vi "2022SignalManipulation.vi"(9 "Cold Junction Temp":dbl, 11 "Data":dbl[][](array[numeric])) -> (3 "Array":dbl[](array[numeric]))   [LabVIEW 2021]
panel:
  out "Array 3":dbl[](array[numeric])
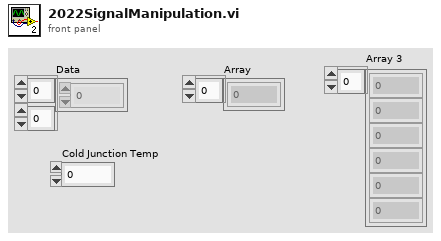
[diagram p1: front panel]
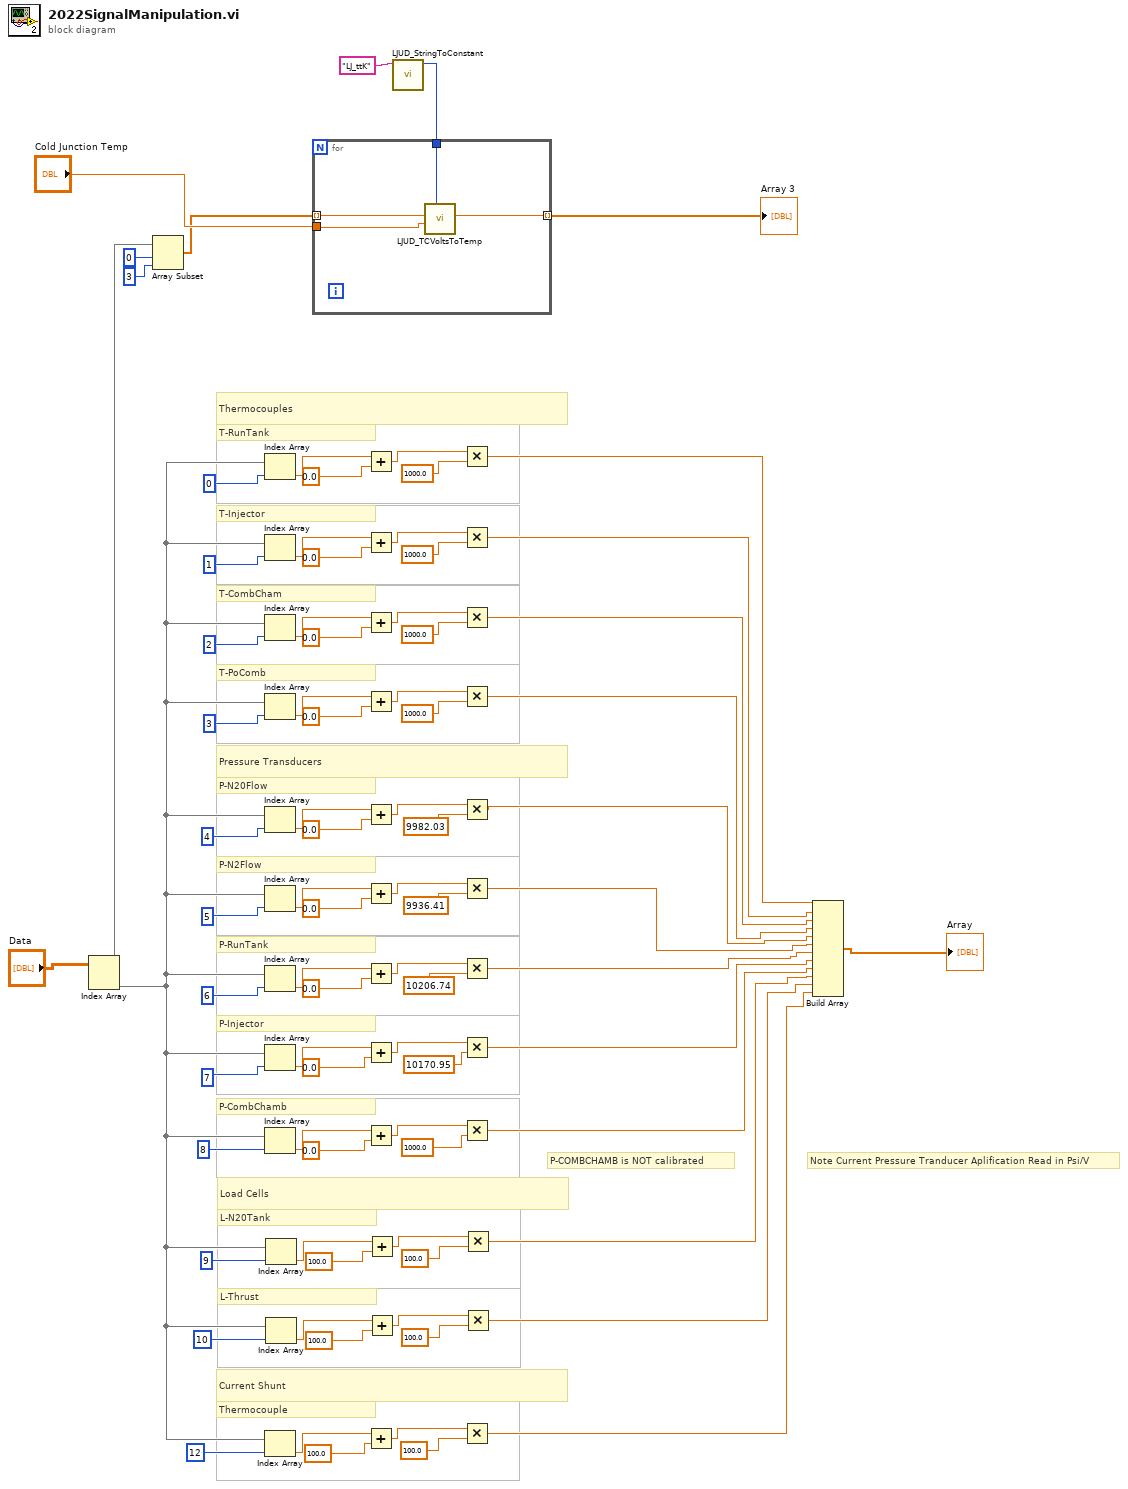
[diagram p0: block diagram]
diagram:
  # "P-COMBCHAMB is NOT calibrated"
  # "Note Current Pressure Tranducer Aplification Read in Psi/V"
  # "L-Thrust"
  # "Load Cells"
  # "L-N20Tank"
  # "P-CombChamb"
  # "Current Shunt"
  # "Thermocouple"
  # "P-Injector"
  # "P-RunTank"
  # "P-N2Flow"
  # "Pressure Transducers"
  # "P-N20Flow"
  # "T-PoComb"
  # "T-CombCham"
  # "T-Injector"
  # "Thermocouples"
  # "T-RunTank"
  n1 = Index Array(array="Data") -> (element=w16:dbl[])  [unwired: 2 in]
  n2 = Array Subset(array=w16, index=0, length=3) -> (w27:dbl[])
  n3 = Index Array(array=w16, index=0 ("index (col)")) -> (element=w57:dbl)
  n4 = Index Array(array=w16, index=1 ("index (col)")) -> (element=w56:dbl)
  n5 = Index Array(array=w16, index=2 ("index (col)")) -> (element=w55:dbl)
  n6 = Index Array(array=w16, index=3 ("index (col)")) -> (element=w54:dbl)
  n7 = Index Array(array=w16, index=4 ("index (col)")) -> (element=w53:dbl)
  n8 = Index Array(array=w16, index=5 ("index (col)")) -> (element=w52:dbl)
  n9 = Index Array(array=w16, index=6 ("index (col)")) -> (element=w51:dbl)
  n10 = Index Array(array=w16, index=7 ("index (col)")) -> (element=w50:dbl)
  n11 = Index Array(array=w16, index=8 ("index (col)")) -> (element=w47:dbl)
  n12 = Index Array(array=w16, index=12 ("index (col)")) -> (element=w44:dbl)
  n13 = Index Array(array=w16, index=9) -> (element=w18:dbl)
  n14 = Index Array(array=w16, index=10) -> (element=w17:dbl)
  n15 = Add(x=w57, y=0.0) -> (x+y=w82:dbl)
  n16 = Add(x=w56, y=0.0) -> (x+y=w79:dbl)
  n17 = Add(x=w55, y=0.0) -> (x+y=w76:dbl)
  n18 = Add(x=w54, y=0.0) -> (x+y=w73:dbl)
  n19 = Add(x=w53, y=0.0) -> (x+y=w70:dbl)
  n20 = Add(x=w52, y=0.0) -> (x+y=w67:dbl)
  n21 = Add(x=w51, y=0.0) -> (x+y=w64:dbl)
  n22 = Add(x=w50, y=0.0) -> (x+y=w61:dbl)
  n23 = Add(x=w47, y=0.0) -> (x+y=w58:dbl)
  n24 = Add(x=w44, y=100.0) -> (x+y=w60:dbl)
  n25 = Add(x=w18, y=100.0) -> (x+y=w24:dbl)
  n26 = Add(x=w17, y=100.0) -> (x+y=w21:dbl)
  n27 = call "LJUD_StringToConstant.vi"("String"="LJ_ttK") -> ("Constant Number"=w25:i32)  [unwired: 9 in, 1 out]
  n28 = for {
    tunnel: "Cold Junction Temp" -> [w85]
    tunnel: w27 -> [w86] mode=indexing
    tunnel: [w83] -> w26 mode=indexing
    tunnel: w25 -> [w84]
    n29 = call "LJUD_TCVoltsToTemp.vi"("TCType"=w84, "CJTempK"=w85, "TCVolts"=w86) -> ("TCTempC"=w83:dbl)  [unwired: 5 in, 3 out]
  }
  "Array 3" <- w26
  n30 = Multiply(x=w82, y=1000.0) -> (x*y=w13:dbl)
  n31 = Multiply(x=w79, y=1000.0) -> (x*y=w12:dbl)
  n32 = Multiply(x=w76, y=1000.0) -> (x*y=w11:dbl)
  n33 = Multiply(x=w73, y=1000.0) -> (x*y=w10:dbl)
  n34 = Multiply(x=w70, y=9982.03) -> (x*y=w9:dbl)
  n35 = Multiply(x=w67, y=9936.41) -> (x*y=w8:dbl)
  n36 = Multiply(x=w64, y=10206.74) -> (x*y=w7:dbl)
  n37 = Multiply(x=w61, y=10170.95) -> (x*y=w6:dbl)
  n38 = Multiply(x=w58, y=1000.0) -> (x*y=w5:dbl)
  n39 = Multiply(x=w60, y=100.0) -> (x*y=w2:dbl)
  n40 = Multiply(x=w24, y=100.0) -> (x*y=w4:dbl)
  n41 = Multiply(x=w21, y=100.0) -> (x*y=w3:dbl)
  n42 = Build Array(w13, w12, w11, w10, w9, w8, w7, w6, w5, w4, w3, w2) -> (→"Array":dbl[])
